vi "Get Plugin Port From Tree Reference.vi"(8 "error in (no error)":errorcluster, 11 "Loaded Plugins":refnum<vi>) -> (0 "error out":errorcluster, 3 "Plugin port":i32)   [LabVIEW 2021, in "CIF_Manager_UI.lvclass"]
uses:
  CIF_Manager_UI.lvclass
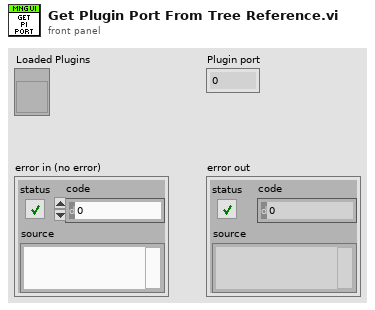
[diagram p1: front panel]
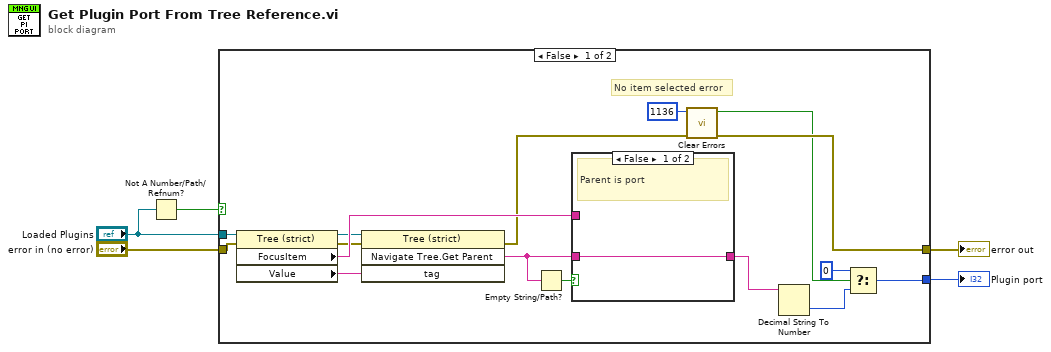
[diagram p0: block diagram]
diagram:
  n1 = Not A Number/Path/Refnum?(number/path/refnum="Loaded Plugins") -> (NaN/Path/Refnum?=w2:bool)
  n2 = case shown="False" w2 {
    tunnel: "error in (no error)" -> [w15 w23]
    tunnel: [w12 w23] -> w4
    tunnel: [w11 _] -> w1
    tunnel: "Loaded Plugins" -> [w9 _]
    frame False {
      # "No item selected error"
      n3 = property class="Tree (strict)"(reference=w9, error in=w15) -> (error out=w16:errorcluster, "FocusItem"=w17:string, "Value"=w20:string)  [unwired: 1 out]
      n4 = invoke class="Tree (strict)" method="Navigate Tree.Get Parent"(reference=w9, error in=w16, "tag"=w20) -> (error out=w13:errorcluster, "Navigate Tree:Get Parent"=w18:string)  [unwired: 1 in, 2 out]
      n5 = Empty String/Path?(string/path=w18) -> (empty?=w19:bool)
      n6 = case shown="False" w19 {
        tunnel: w18 -> [w21 _]
        tunnel: w17 -> [_ w22]
        tunnel: [w21 w22] -> w8
        frame False {
          # "Parent is port"
        }
        frame True {
          # "No parent, item is port"
        }
      }
      n7 = call <vilib>:"Clear Errors.vi"("error in (no error)"=w13, "specific error code to clear (0: all)"=1136) -> ("error out"=w12:errorcluster, "specific error cleared?"=w10:bool)  [unwired: 4 in]
      n8 = Decimal String To Number(string=w8) -> (number=w7:i32)  [unwired: 2 in, 1 out]
      n9 = Select(t=0, s=w10, f=w7) -> (s? t:f=w11:i32)
    }
    frame True {
    }
  }
  "error out" <- w4
  "Plugin port" <- w1
